vi "Configure Display.vi"(0 "VISA resource name":refnum<visa-resource-name>, 1 "Softkey Label (T: Enable)":bool=TRUE, 3 "Frequency (T: Enable)":bool=TRUE, 4 "Display Type (0: Normal)":u16(ring) items=["Normal", "Invert"], 5 "Statistic Analysis Result (F: Disable)":bool, 7 "error in (no error)":errorcluster, 8 "Channel (1)":i32=1, 9 "Graticule Label (T: Enable)":bool=TRUE, 12 "Backlight (T: Enable)":bool=TRUE, 13 "Table Type (0: Marker table)":u16(ring) items=["Marker table", "Limit test table", "Segment table", " Echo window", "Loss comp. table", "Power sensor (SC Factor)", "Ripple test"], 14 "Display Update (T: Enable)":bool=TRUE, 15 "Title Text (\"Title\")":string="Title", 16 "Clock (T: Enable)":bool=TRUE, 17 "Table (F: Disable)":bool, 19 "Maximization (F: Off)":bool) -> (20 "VISA resource name out":refnum<visa-resource-name>, 27 "error out":errorcluster)   [LabVIEW 2011, in "Agilent ENA Series.lvlib"]
doc: "This VI configures display paramters."
uses:
  Agilent ENA Series.lvlib
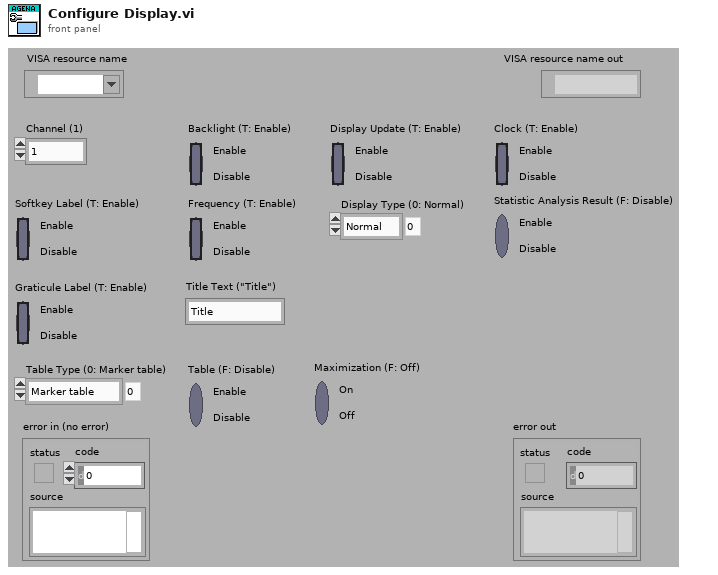
[diagram p1: front panel]
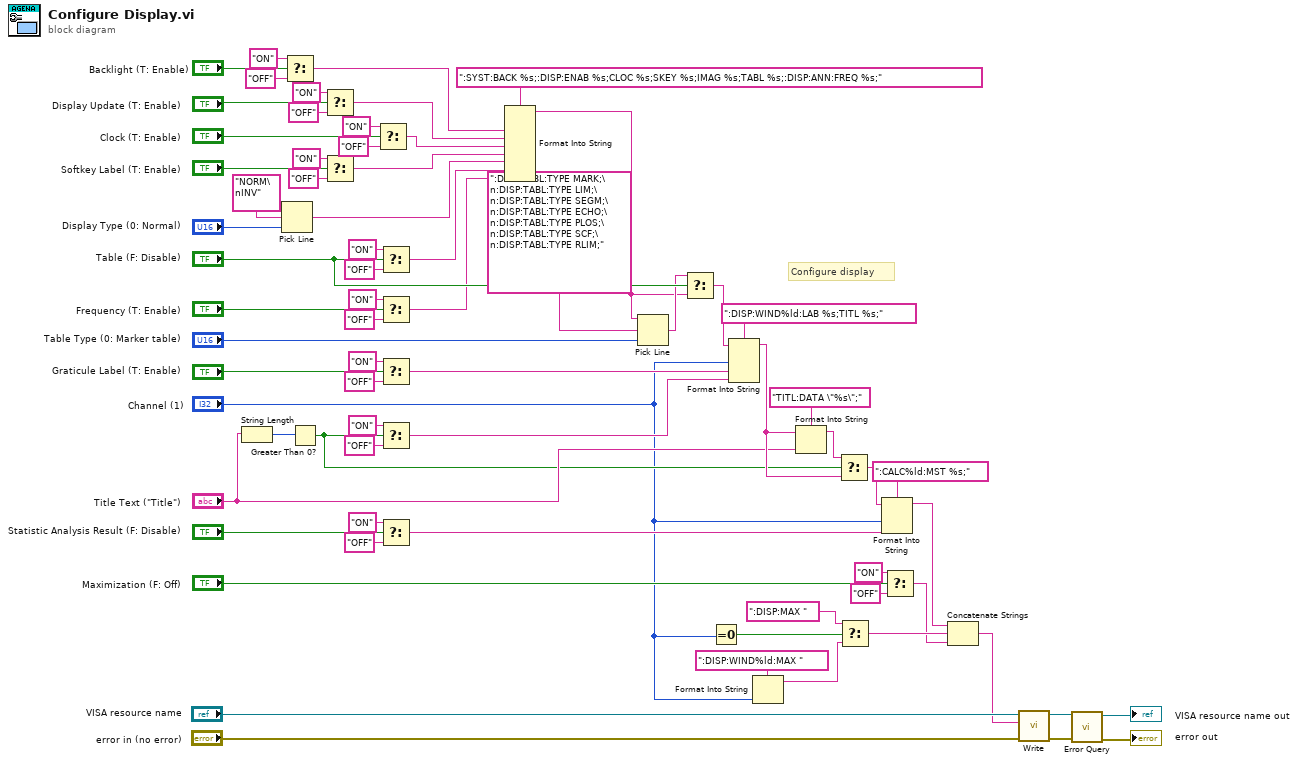
[diagram p0: block diagram]
diagram:
  # "Configure display"
  n1 = String Length(string="Title Text (\"Title\")") -> (length=w14:i32)
  n2 = Pick Line(multi-line string="NORM\nINV", line index="Display Type (0: Normal)") -> (output string=w50:string)  [unwired: 1 in]
  n3 = Select(t="ON", s="Backlight (T: Enable)", f="OFF") -> (s? t:f=w62:string)
  n4 = Greater Than 0?(x=w14) -> (x > 0?=w13:bool)
  n5 = Select(t="ON", s="Display Update (T: Enable)", f="OFF") -> (s? t:f=w61:string)
  n6 = Select(t="ON", s="Softkey Label (T: Enable)", f="OFF") -> (s? t:f=w53:string)
  n7 = Select(t="ON", s="Clock (T: Enable)", f="OFF") -> (s? t:f=w57:string)
  n8 = Select(t="ON", s="Table (F: Disable)", f="OFF") -> (s? t:f=w47:string)
  n9 = Select(t="ON", s="Frequency (T: Enable)", f="OFF") -> (s? t:f=w20:string)
  n10 = Select(t="ON", s="Graticule Label (T: Enable)", f="OFF") -> (s? t:f=w37:string)
  n11 = Select(t="ON", s=w13, f="OFF") -> (s? t:f=w34:string)
  n12 = Select(t="ON", s="Statistic Analysis Result (F: Disable)", f="OFF") -> (s? t:f=w28:string)
  n13 = Format Into String(format string=":SYST:BACK %s;:DISP:ENAB %s;CLOC %s;SKEY %s;IMAG %s;TABL %s;:DISP:ANN:FREQ %s;", w62, w61, w57, w53, w50, w47, w20) -> (resulting string=w27:string)  [unwired: 2 in, 1 out]
  n14 = Pick Line(string ("")=w27, multi-line string=":DISP:TABL:TYPE MARK;\n:DISP:TABL:TYPE LIM;\n:DISP:TABL:TYPE SEGM;\n:DISP:TABL:TYPE ECHO;\n:DISP:TABL:TYPE PLOS;\n:DISP:TABL:TYPE SCF;\n:DISP:TABL:TYPE RLIM;", line index="Table Type (0: Marker table)") -> (output string=w43:string)
  n15 = Select(t=w43, s="Table (F: Disable)", f=w27) -> (s? t:f=w39:string)
  n16 = Equal To 0?(x="Channel (1)") -> (x = 0?=w12:bool)
  n17 = Format Into String(format string=":DISP:WIND%ld:LAB %s;TITL %s;", initial string=w39, "Channel (1)", w37, w34) -> (resulting string=w25:string)  [unwired: 1 in, 1 out]
  n18 = Format Into String(format string=":DISP:WIND%ld:MAX ", "Channel (1)") -> (resulting string=w10:string)  [unwired: 2 in, 1 out]
  n19 = Format Into String(format string="TITL:DATA \"%s\";", initial string=w25, "Title Text (\"Title\")") -> (resulting string=w24:string)  [unwired: 1 in, 1 out]
  n20 = Select(t=w24, s=w13, f=w25) -> (s? t:f=w33:string)
  n21 = Select(t=":DISP:MAX ", s=w12, f=w10) -> (s? t:f=w5:string)
  n22 = Format Into String(format string=":CALC%ld:MST %s;", initial string=w33, "Channel (1)", w28) -> (resulting string=w3:string)  [unwired: 1 in, 1 out]
  n23 = Select(t="ON", s="Maximization (F: Off)", f="OFF" ("t")) -> (s? t:f=w4:string)
  n24 = Concatenate Strings(w3, w5, w4) -> (w2:string)
  n25 = call "Write.vi"("error in (no error)"="error in (no error)", "String ()"=w2, "VISA resource name"="VISA resource name") -> ("error out"=w18:errorcluster, "VISA resource name out"=w19:refnum<visa-resource-name>)  [unwired: 6 in, 1 out]
  n26 = call "Error Query.vi"("error in (no error)"=w18, "VISA resource name"=w19) -> ("error out"=→"error out":errorcluster, "VISA resource name out"=→"VISA resource name out":refnum<visa-resource-name>)  [unwired: 6 in, 2 out]
